vi "判定参数.vi"() -> ()   [LabVIEW 2020]
panel:
  in  "逆向空载判定参数":T1
  out "振动判定长度":i32
  out "力特性判定长度":i32[](array[numeric])
  out "电流特性判定长度":i32[](array[numeric])
  out "传感器特性判定长度":i32
  out "逆向空载判定长度":i32
  out "功能判定长度":i32
  out "空载判定长度":i32
  in  "振动判定":T2
  in  "振动判定范围":T3
  in  "电流特性判定参数":T4(array[cluster])
  in  "力特性判定参数":T5(array[cluster])
  in  "功能判定参数":T6
  in  "空载判定参数":T7
  in  "传感器特性判定参数":T8
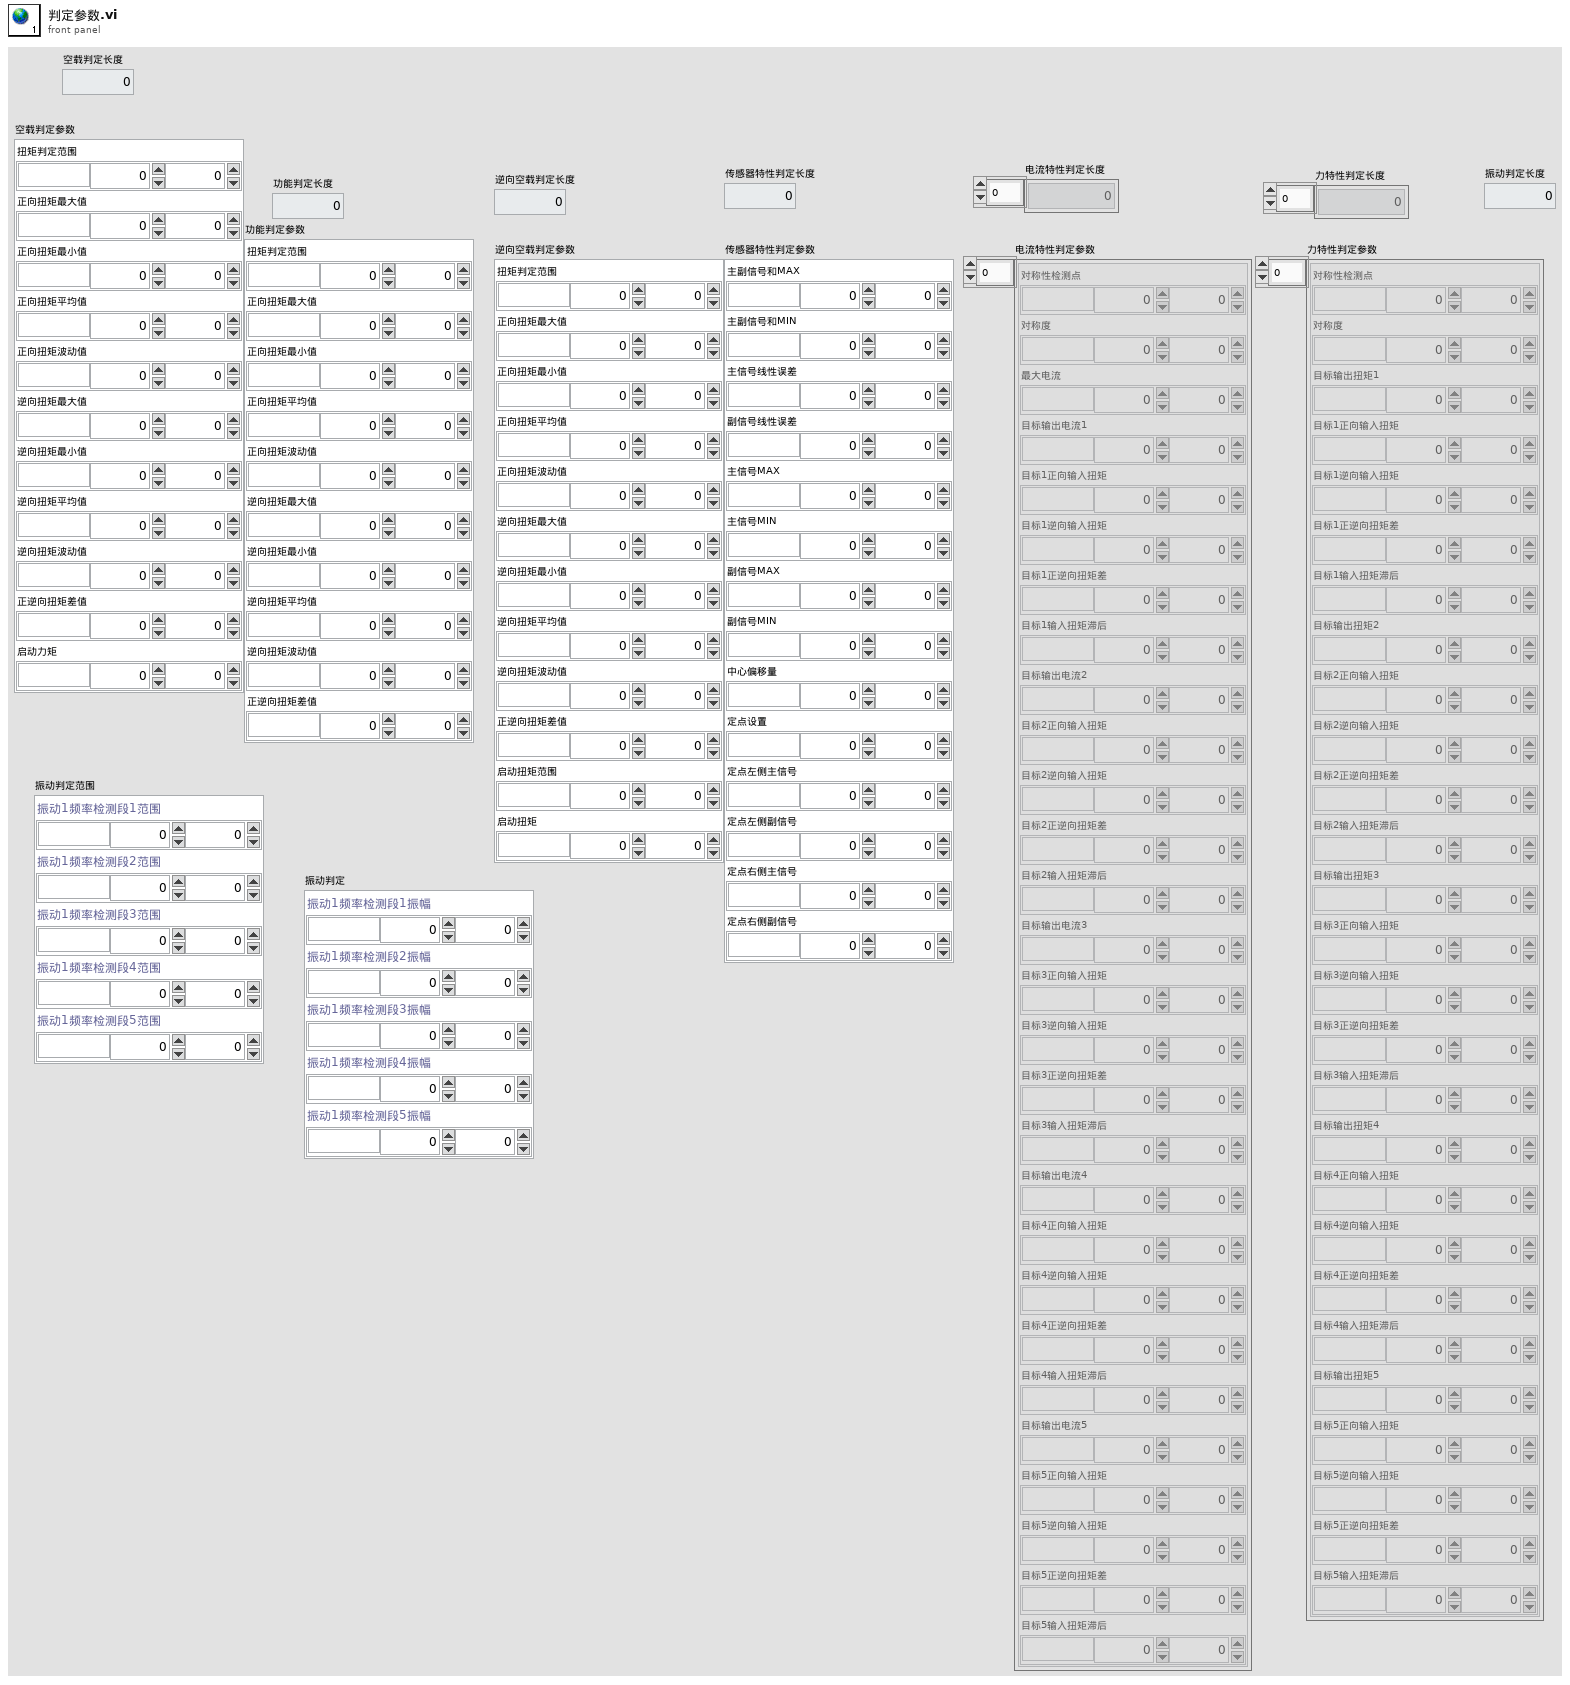
[diagram p1: front panel]
types:
  T1 = cluster{"扭矩判定范围":cluster{"单位":string, "下限":dbl, "上限":dbl}, "正向扭矩最大值":cluster{"单位":string, "下限":dbl, "上限":dbl}, "正向扭矩最小值":cluster{"单位":string, "下限":dbl, "上限":dbl}, "正向扭矩平均值":cluster{"单位":string, "下限":dbl, "上限":dbl}, "正向扭矩波动值":cluster{"单位":string, "下限":dbl, "上限":dbl}, "逆向扭矩最大值":cluster{"单位":string, "下限":dbl, "上限":dbl}, "逆向扭矩最小值":cluster{"单位":string, "下限":dbl, "上限":dbl}, "逆向扭矩平均值":cluster{"单位":string, "下限":dbl, "上限":dbl}, "逆向扭矩波动值":cluster{"单位":string, "下限":dbl, "上限":dbl}, "正逆向扭矩差值":cluster{"单位":string, "下限":dbl, "上限":dbl}, "启动扭矩范围":cluster{"单位":string, "下限":dbl, "上限":dbl}, "启动扭矩":cluster{"单位":string, "下限":dbl, "上限":dbl}}
  T2 = cluster{"振动1频率检测段1振幅":cluster{"单位":string, "下限":dbl, "上限":dbl}, "振动1频率检测段2振幅":cluster{"单位":string, "下限":dbl, "上限":dbl}, "振动1频率检测段3振幅":cluster{"单位":string, "下限":dbl, "上限":dbl}, "振动1频率检测段4振幅":cluster{"单位":string, "下限":dbl, "上限":dbl}, "振动1频率检测段5振幅":cluster{"单位":string, "下限":dbl, "上限":dbl}}
  T3 = cluster{"振动1频率检测段1范围":cluster{"单位":string, "下限":dbl, "上限":dbl}, "振动1频率检测段2范围":cluster{"单位":string, "下限":dbl, "上限":dbl}, "振动1频率检测段3范围":cluster{"单位":string, "下限":dbl, "上限":dbl}, "振动1频率检测段4范围":cluster{"单位":string, "下限":dbl, "上限":dbl}, "振动1频率检测段5范围":cluster{"单位":string, "下限":dbl, "上限":dbl}}
  T4 = cluster{"对称性检测点":cluster{"单位":string, "下限":dbl, "上限":dbl}, "对称度":cluster{"单位":string, "下限":dbl, "上限":dbl}, "最大电流":cluster{"单位":string, "下限":dbl, "上限":dbl}, "目标输出电流1":cluster{"单位":string, "下限":dbl, "上限":dbl}, "目标1正向输入扭矩":cluster{"单位":string, "下限":dbl, "上限":dbl}, "目标1逆向输入扭矩":cluster{"单位":string, "下限":dbl, "上限":dbl}, "目标1正逆向扭矩差":cluster{"单位":string, "下限":dbl, "上限":dbl}, "目标1输入扭矩滞后":cluster{"单位":string, "下限":dbl, "上限":dbl}, "目标输出电流2":cluster{"单位":string, "下限":dbl, "上限":dbl}, "目标2正向输入扭矩":cluster{"单位":string, "下限":dbl, "上限":dbl}, "目标2逆向输入扭矩":cluster{"单位":string, "下限":dbl, "上限":dbl}, "目标2正逆向扭矩差":cluster{"单位":string, "下限":dbl, "上限":dbl}, "目标2输入扭矩滞后":cluster{"单位":string, "下限":dbl, "上限":dbl}, "目标输出电流3":cluster{"单位":string, "下限":dbl, "上限":dbl}, "目标3正向输入扭矩":cluster{"单位":string, "下限":dbl, "上限":dbl}, "目标3逆向输入扭矩":cluster{"单位":string, "下限":dbl, "上限":dbl}, "目标3正逆向扭矩差":cluster{"单位":string, "下限":dbl, "上限":dbl}, "目标3输入扭矩滞后":cluster{"单位":string, "下限":dbl, "上限":dbl}, "目标输出电流4":cluster{"单位":string, "下限":dbl, "上限":dbl}, "目标4正向输入扭矩":cluster{"单位":string, "下限":dbl, "上限":dbl}, "目标4逆向输入扭矩":cluster{"单位":string, "下限":dbl, "上限":dbl}, "目标4正逆向扭矩差":cluster{"单位":string, "下限":dbl, "上限":dbl}, "目标4输入扭矩滞后":cluster{"单位":string, "下限":dbl, "上限":dbl}, "目标输出电流5":cluster{"单位":string, "下限":dbl, "上限":dbl}, "目标5正向输入扭矩":cluster{"单位":string, "下限":dbl, "上限":dbl}, "目标5逆向输入扭矩":cluster{"单位":string, "下限":dbl, "上限":dbl}, "目标5正逆向扭矩差":cluster{"单位":string, "下限":dbl, "上限":dbl}, "目标5输入扭矩滞后":cluster{"单位":string, "下限":dbl, "上限":dbl}}[]
  T5 = cluster{"对称性检测点":cluster{"单位":string, "下限":dbl, "上限":dbl}, "对称度":cluster{"单位":string, "下限":dbl, "上限":dbl}, "目标输出扭矩1":cluster{"单位":string, "下限":dbl, "上限":dbl}, "目标1正向输入扭矩":cluster{"单位":string, "下限":dbl, "上限":dbl}, "目标1逆向输入扭矩":cluster{"单位":string, "下限":dbl, "上限":dbl}, "目标1正逆向扭矩差":cluster{"单位":string, "下限":dbl, "上限":dbl}, "目标1输入扭矩滞后":cluster{"单位":string, "下限":dbl, "上限":dbl}, "目标输出扭矩2":cluster{"单位":string, "下限":dbl, "上限":dbl}, "目标2正向输入扭矩":cluster{"单位":string, "下限":dbl, "上限":dbl}, "目标2逆向输入扭矩":cluster{"单位":string, "下限":dbl, "上限":dbl}, "目标2正逆向扭矩差":cluster{"单位":string, "下限":dbl, "上限":dbl}, "目标2输入扭矩滞后":cluster{"单位":string, "下限":dbl, "上限":dbl}, "目标输出扭矩3":cluster{"单位":string, "下限":dbl, "上限":dbl}, "目标3正向输入扭矩":cluster{"单位":string, "下限":dbl, "上限":dbl}, "目标3逆向输入扭矩":cluster{"单位":string, "下限":dbl, "上限":dbl}, "目标3正逆向扭矩差":cluster{"单位":string, "下限":dbl, "上限":dbl}, "目标3输入扭矩滞后":cluster{"单位":string, "下限":dbl, "上限":dbl}, "目标输出扭矩4":cluster{"单位":string, "下限":dbl, "上限":dbl}, "目标4正向输入扭矩":cluster{"单位":string, "下限":dbl, "上限":dbl}, "目标4逆向输入扭矩":cluster{"单位":string, "下限":dbl, "上限":dbl}, "目标4正逆向扭矩差":cluster{"单位":string, "下限":dbl, "上限":dbl}, "目标4输入扭矩滞后":cluster{"单位":string, "下限":dbl, "上限":dbl}, "目标输出扭矩5":cluster{"单位":string, "下限":dbl, "上限":dbl}, "目标5正向输入扭矩":cluster{"单位":string, "下限":dbl, "上限":dbl}, "目标5逆向输入扭矩":cluster{"单位":string, "下限":dbl, "上限":dbl}, "目标5正逆向扭矩差":cluster{"单位":string, "下限":dbl, "上限":dbl}, "目标5输入扭矩滞后":cluster{"单位":string, "下限":dbl, "上限":dbl}}[]
  T6 = cluster{"扭矩判定范围":cluster{"单位":string, "下限":dbl, "上限":dbl}, "正向扭矩最大值":cluster{"单位":string, "下限":dbl, "上限":dbl}, "正向扭矩最小值":cluster{"单位":string, "下限":dbl, "上限":dbl}, "正向扭矩平均值":cluster{"单位":string, "下限":dbl, "上限":dbl}, "正向扭矩波动值":cluster{"单位":string, "下限":dbl, "上限":dbl}, "逆向扭矩最大值":cluster{"单位":string, "下限":dbl, "上限":dbl}, "逆向扭矩最小值":cluster{"单位":string, "下限":dbl, "上限":dbl}, "逆向扭矩平均值":cluster{"单位":string, "下限":dbl, "上限":dbl}, "逆向扭矩波动值":cluster{"单位":string, "下限":dbl, "上限":dbl}, "正逆向扭矩差值":cluster{"单位":string, "下限":dbl, "上限":dbl}}
  T7 = cluster{"扭矩判定范围":cluster{"单位":string, "下限":dbl, "上限":dbl}, "正向扭矩最大值":cluster{"单位":string, "下限":dbl, "上限":dbl}, "正向扭矩最小值":cluster{"单位":string, "下限":dbl, "上限":dbl}, "正向扭矩平均值":cluster{"单位":string, "下限":dbl, "上限":dbl}, "正向扭矩波动值":cluster{"单位":string, "下限":dbl, "上限":dbl}, "逆向扭矩最大值":cluster{"单位":string, "下限":dbl, "上限":dbl}, "逆向扭矩最小值":cluster{"单位":string, "下限":dbl, "上限":dbl}, "逆向扭矩平均值":cluster{"单位":string, "下限":dbl, "上限":dbl}, "逆向扭矩波动值":cluster{"单位":string, "下限":dbl, "上限":dbl}, "正逆向扭矩差值":cluster{"单位":string, "下限":dbl, "上限":dbl}, "启动力矩":cluster{"单位":string, "下限":dbl, "上限":dbl}}
  T8 = cluster{"主副信号和MAX":cluster{"单位":string, "下限":dbl, "上限":dbl}, "主副信号和MIN":cluster{"单位":string, "下限":dbl, "上限":dbl}, "主信号线性误差":cluster{"单位":string, "下限":dbl, "上限":dbl}, "副信号线性误差":cluster{"单位":string, "下限":dbl, "上限":dbl}, "主信号MAX":cluster{"单位":string, "下限":dbl, "上限":dbl}, "主信号MIN":cluster{"单位":string, "下限":dbl, "上限":dbl}, "副信号MAX":cluster{"单位":string, "下限":dbl, "上限":dbl}, "副信号MIN":cluster{"单位":string, "下限":dbl, "上限":dbl}, "中心偏移量":cluster{"单位":string, "下限":dbl, "上限":dbl}, "定点设置":cluster{"单位":string, "下限":dbl, "上限":dbl}, "定点左侧主信号":cluster{"单位":string, "下限":dbl, "上限":dbl}, "定点左侧副信号":cluster{"单位":string, "下限":dbl, "上限":dbl}, "定点右侧主信号":cluster{"单位":string, "下限":dbl, "上限":dbl}, "定点右侧副信号":cluster{"单位":string, "下限":dbl, "上限":dbl}}
diagram:
